vi "Host_PC.vi"() -> ()   [LabVIEW 2011, in "Brian.lvrbt"]
uses:
  <vilib>/NXT/NXT Controls/ConnectionType.ctl
  Brian.lvrbt
panel:
  out "NXT Seconds Elapsed":string="0"
  in  "Connection type":T1
  in  "NXT name":string="MyNXT"
  in  "Speed":i32(knob)=1 caption="Message" scale=-100.0..100.0
  out "Is Paired?":bool
  in  "stop":bool
  # "Steps:\n1. Connect NXT Motor NXT Port A\n2. Download and run Client_NXT.vi on the NXT.\n3. Set NXT Name and Connection Type appropriately on this VI.\n4. Run this VI.\n5. Use the Speed dial to adjust the motor speed on the NXT."
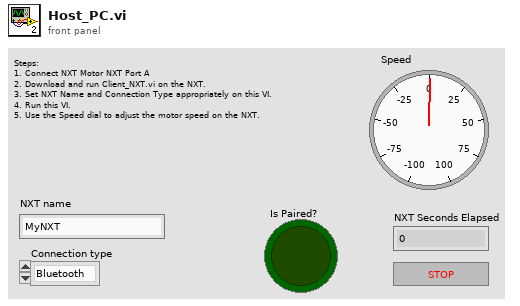
[diagram p1: front panel]
types:
  T1 = typedef "ConnectionType.ctl" = enum16{"Bluetooth", "USB", "WiFi"}
  T2 = typedef "nxt.ctl" = cluster{"nxtHandle":u32, "fileHandle":u32, "fileIterHandle":u32, "moduleHandle":u32, "modIterHandle":u32, "nxtIterHandle":u32}
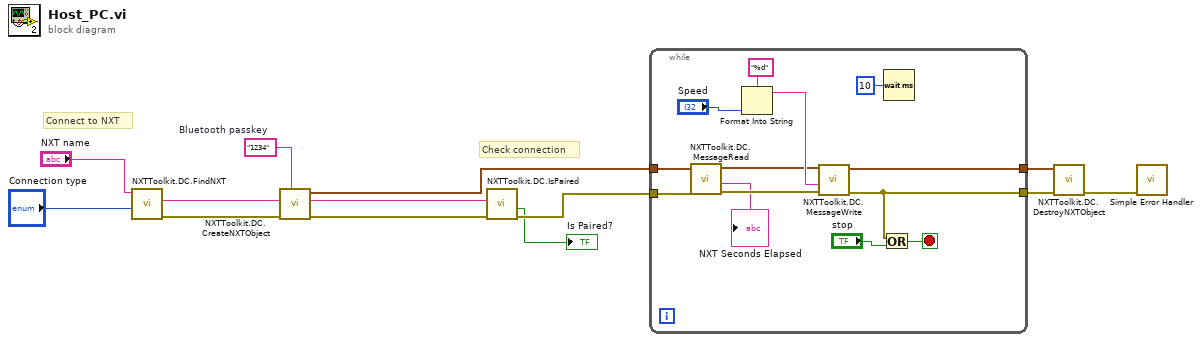
[diagram p0: block diagram]
diagram:
  w10 = "1234"  # Bluetooth passkey
  # "Check connection"
  # "Connect to NXT"
  n1 = call <vilib>:"NXTToolkit.DC.FindNXT.vi"("Connection type (USB)"="Connection type", "NXT name"="NXT name") -> ("error out"=w9:errorcluster, "VISA resource string"=w8:string)  [unwired: 7 in, 1 out]
  n2 = call <vilib>:"NXTToolkit.DC.CreateNXTObject.vi"("Bluetooth passkey (1234)"=w10, "error in (no error)"=w9, "VISA resource string (\"\" : find USB brick)"=w8) -> ("error out"=w7:errorcluster, "VISA resource string out"=w6:string, "NXTObject"=w4:T2)  [unwired: 6 in]
  n3 = call <vilib>:"NXTToolkit.DC.IsPaired.vi"("error in (no error)"=w7, "VISA resource string"=w6) -> ("error out"=w3:errorcluster, "Is Paired?"=→"Is Paired?":bool)  [unwired: 7 in, 1 out]
  n4 = while {
    tunnel: w3 -> [w16]
    tunnel: [w19] -> w12
    tunnel: w4 -> [w18]
    tunnel: [w20] -> w11
    stop <- w24 stop-if-true
    n5 = call <vilib>:"NXTToolkit.DC.MessageRead.vi"("error in (no error)"=w16, "NXTObject"=w18) -> ("error out"=w15:errorcluster, "Message"=→"NXT Seconds Elapsed":string, "NXTObject dup"=w17:T2)  [unwired: 4 in, 3 out]
    n6 = Format Into String(format string="%d", "Speed") -> (resulting string=w22:string)  [unwired: 2 in, 1 out]
    n7 = call <vilib>:"NXTToolkit.DC.MessageWrite.vi"("error in (no error)"=w15, "Message"=w22, "NXTObject"=w17) -> ("error out"=w19:errorcluster, "NXTObject dup"=w20:T2)  [unwired: 5 in, 2 out]
    n8 = Or(x=w19, y="stop") -> (x .or. y?=w24:bool)
    n9 = Wait (ms)(milliseconds to wait=u32 10) -> ()  [unwired: 1 out]
  }
  n10 = call <vilib>:"NXTToolkit.DC.DestroyNXTObject.vi"("error in (no error)"=w12, "NXTObject"=w11) -> ("error out"=w13:errorcluster)  [unwired: 9 in]
  n11 = call <vilib>:"Simple Error Handler.vi"("error in (no error)"=w13) -> ()  [unwired: 4 in, 5 out]
